vi "Basic Get Instruments Info.vi"() -> ()   [LabVIEW 2016]
doc: "Purpose: This example shows how to retrieve information about Fluigent instruments: type, controller, serial number, unique ID...\nHardware setup: At least one Fluigent pressure or sensor module"
uses:
  TypeDefs/fgt_INSTRUMENT_TYPE.ctl
  TypeDefs/fgt_CHANNEL_INFO.ctl
  TypeDefs/fgt_SENSOR_TYPE.ctl
  TypeDefs/fgt_CONTROLLER_INFO.ctl
  TypeDefs/fgt_VALVE_TYPE.ctl
  fgt_SDK.lvlib
panel:
  in  "Tab Control":T1(tab)
  out "Controllers channels info":T2[](array[typedef]) {"firmware" format="%04x"}
  out "Detected instruments":T4(array[cluster])
  out "Controllers count":i32
  out "Instruments count":i32
  out "Valve channels type":T5[](array[typedef])
  out "Valve channels count":u32
  out "Valve channels info":T6[](array[typedef]) {"firmware" format="%04x"}
  out "Pressure channels count":u32
  out "Sensor channels count":u32
  out "TTL channels count":u32
  out "Pressure channels info":T6[](array[typedef]) {"firmware" format="%04x"}
  out "Sensor channels info":T6[](array[typedef]) {"firmware" format="%04x"}
  out "Sensor channels type":T7[](array[typedef])
  out "TTL channels info":T6[](array[typedef]) {"firmware" format="%04x"}
  out "error out":errorcluster
  # "Hit the \"Run\" button to retrieve information about all Fluigent connected instruments"
  # "Hit the \"Run\" button to start the regulation"
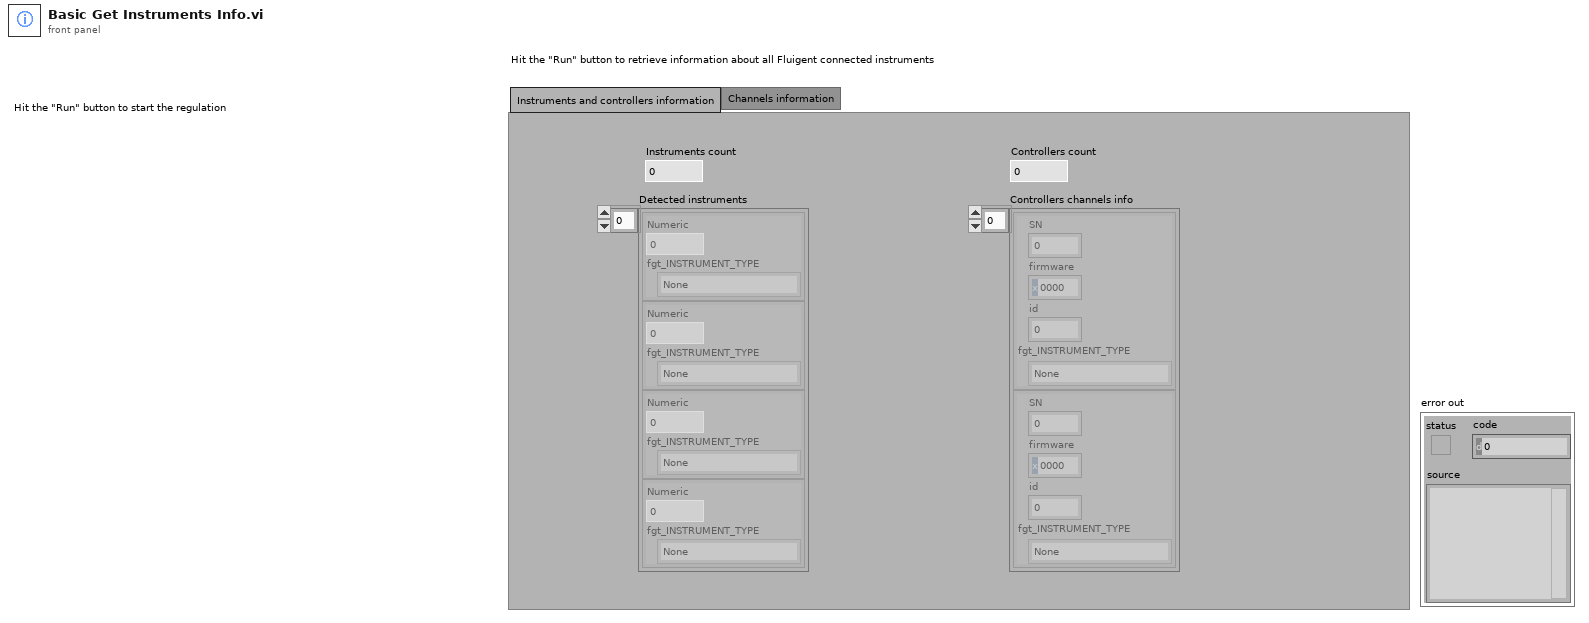
[diagram p1: front panel]
types:
  T1 = enum32{"Instruments and controllers information", "Channels information"}
  T2 = typedef "fgt_SDK.lvlib/fgt_CONTROLLER_INFO.ctl" = cluster{"SN":u16, "firmware":u16, "id":u32, "fgt_INSTRUMENT_TYPE":T3}
  T3 = typedef "fgt_SDK.lvlib/fgt_INSTRUMENT_TYPE.ctl" = enum32{"None", "MFCS", "MFCS_EZ", "FRP", "LineUP", "IPS"}
  T4 = cluster{"Numeric":u16, "fgt_INSTRUMENT_TYPE":T3}[]
  T5 = typedef "fgt_SDK.lvlib/fgt_VALVE_TYPE.ctl" = enum32{"None", "MSwitch", "TwoSwitch", "LSwitch", "PSwitch"}
  T6 = typedef "fgt_SDK.lvlib/fgt_CHANNEL_INFO.ctl" = cluster{"ControllerSN":u16, "firmware":u16, "DeviceSN":u16, "position":u32, "index":u32, "indexID":u32, "fgt_INSTRUMENT_TYPE":T3}
  T7 = typedef "fgt_SDK.lvlib/fgt_SENSOR_TYPE.ctl" = enum32{"None", "XS_single", "S_single", "S_dual", "M_single", "M_dual", "L_single", "L_dual", "XL_single", "Pressure_S", "Pressure_M", "Pressure_XL"}
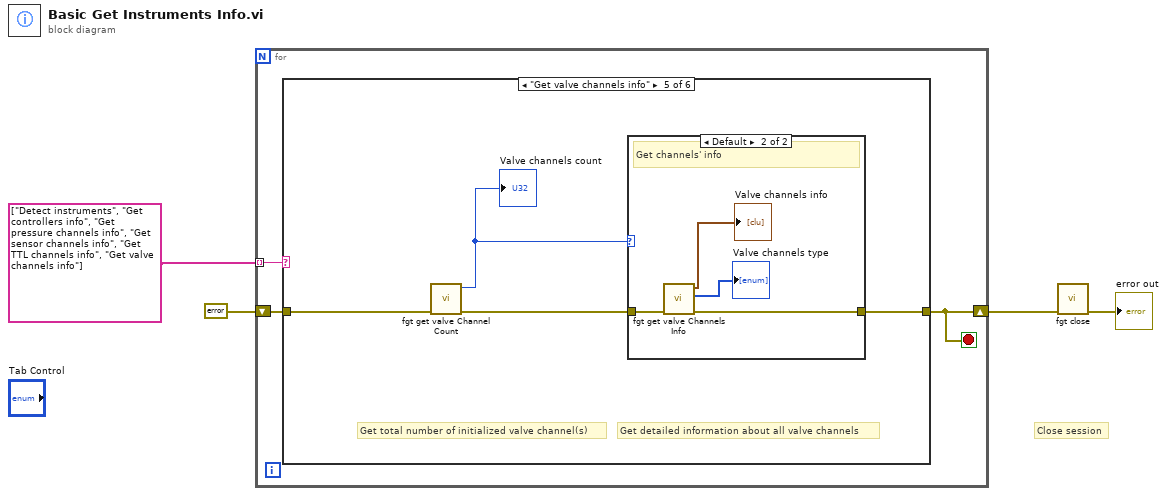
[diagram p0: block diagram]
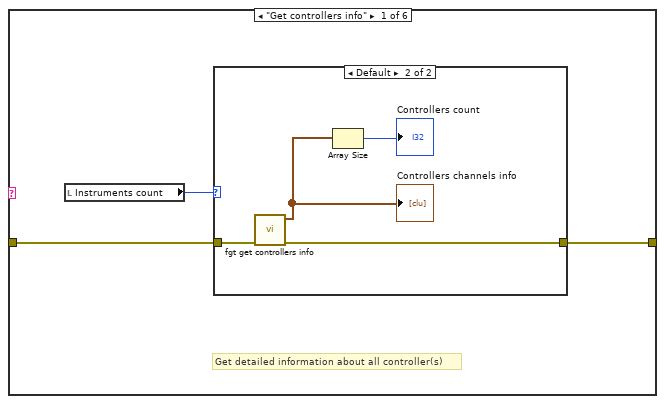
[diagram p2: hidden frame]
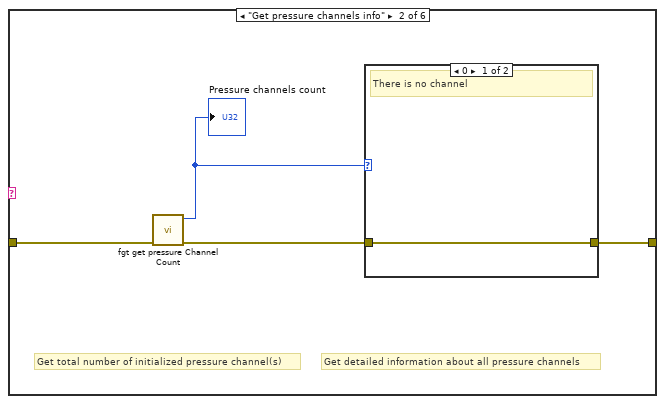
[diagram p4: hidden frame]
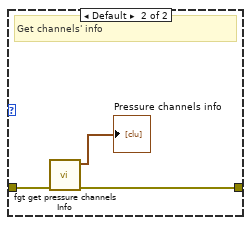
[diagram p5: hidden frame]
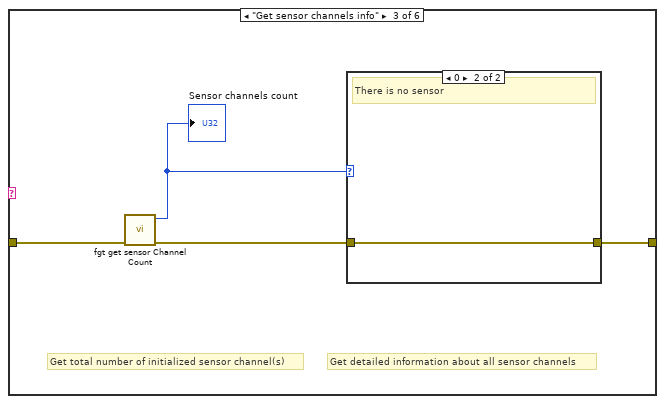
[diagram p6: hidden frame]
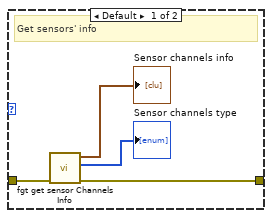
[diagram p7: hidden frame]
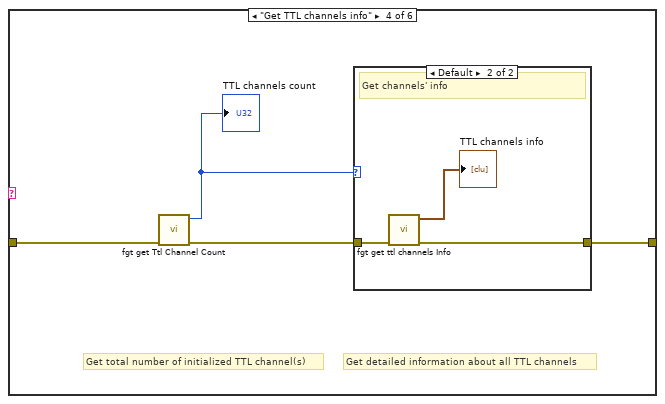
[diagram p8: hidden frame]
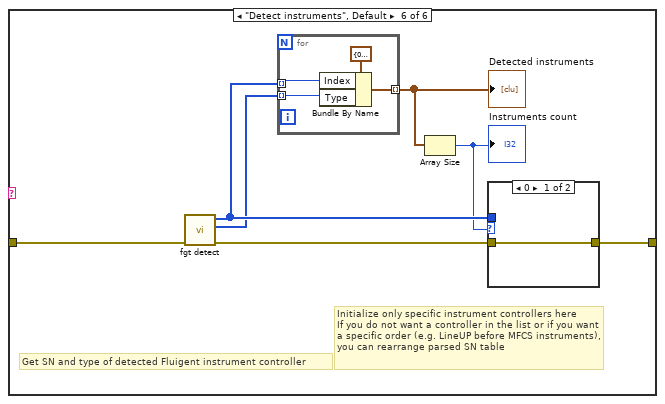
[diagram p11: hidden frame]
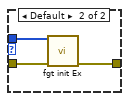
[diagram p12: hidden frame]
diagram:
  # "Close session"
  n1 = for {
    tunnel: string[] ["Detect instruments", "Get controllers info", "Get pressure channels info", "Get sensor channels info", "Get TTL channels info", "Get valve channels info"] -> [w7] mode=indexing
    shift-right: [w5] -> w1
    shift-left: errorcluster {"status"=FALSE, "code"=0, "source"=""} ("error in (no error)") -> [w6]
    stop <- w5 stop-if-true
    n2 = case shown="\"Get valve channels info\"" w7 {
      tunnel: [w9 w17 w25 w34 w44 w53] -> w5
      tunnel: w6 -> [w10 w18 w26 w35 w43 w52]
      frame "Get controllers info" {
        # "Get detailed information about all controller(s)"
        n3 = local read "Instruments count"() -> (w8:i32)
        n4 = case shown="Default" w8 {
          tunnel: w10 -> [w11 w15]
          tunnel: [w11 w14] -> w9
          frame 0 {
          }
          frame Default {
            n5 = call "fgt get controllers info.vi"("error in (no error)"=w15) -> ("error out"=w14:errorcluster, "Controllers channels info"=w12:T2[])  [unwired: 9 in]
            "Controllers channels info" <- w12
            n6 = Array Size(array=w12) -> (size(s)=→"Controllers count":i32)
          }
        }
      }
      frame "Get pressure channels info" {
        # "Get detailed information about all pressure channels"
        # "Get total number of initialized pressure channel(s)"
        n7 = call "fgt get pressure Channel Count.vi"("error in (no error)"=w18) -> ("error out"=w19:errorcluster, "nbPChan out"=w16:u32)  [unwired: 9 in]
        "Pressure channels count" <- w16
        n8 = case shown="0" w16 {
          tunnel: w19 -> [w20 w22]
          tunnel: [w20 w21] -> w17
          frame 0 {
            # "There is no channel"
          }
          frame Default {
            # "Get channels' info"
            n9 = call "fgt get pressure channels Info.vi"("error in (no error)"=w22) -> ("error out"=w21:errorcluster, "Pressure channels info"=→"Pressure channels info":T6[])  [unwired: 9 in]
          }
        }
      }
      frame "Get sensor channels info" {
        # "Get detailed information about all sensor channels"
        # "Get total number of initialized sensor channel(s)"
        n10 = call "fgt get sensor Channel Count.vi"("error in (no error)"=w26) -> ("error out"=w27:errorcluster, "nbSChan out"=w24:u32)  [unwired: 9 in]
        "Sensor channels count" <- w24
        n11 = case shown="0" w24 {
          tunnel: w27 -> [w29 w32]
          tunnel: [w28 w32] -> w25
          frame Default {
            # "Get sensors' info"
            n12 = call "fgt get sensor Channels Info.vi"("error in (no error)"=w29) -> ("error out"=w28:errorcluster, "Sensor channels type"=→"Sensor channels type":T7[], "Sensor channels info"=→"Sensor channels info":T6[])  [unwired: 8 in]
          }
          frame 0 {
            # "There is no sensor"
          }
        }
      }
      frame "Get TTL channels info" {
        # "Get detailed information about all TTL channels"
        # "Get total number of initialized TTL channel(s)"
        n13 = call "fgt get Ttl Channel Count.vi"("error in (no error)"=w35) -> ("error out"=w36:errorcluster, "nbTtlChan out"=w33:u32)  [unwired: 9 in]
        "TTL channels count" <- w33
        n14 = case shown="Default" w33 {
          tunnel: w36 -> [w37 w39]
          tunnel: [w37 w38] -> w34
          frame 0 {
            # "There is no channel"
          }
          frame Default {
            # "Get channels' info"
            n15 = call "fgt get ttl channels Info.vi"("error in (no error)"=w39) -> ("error out"=w38:errorcluster, "TTL channels info"=→"TTL channels info":T6[])  [unwired: 9 in]
          }
        }
      }
      frame "Get valve channels info" {
        # "Get detailed information about all valve channels"
        # "Get total number of initialized valve channel(s)"
        n16 = call "fgt get valve Channel Count.vi"("error in (no error)"=w43) -> ("error out"=w42:errorcluster, "nbVChan out"=w41:u32)  [unwired: 9 in]
        "Valve channels count" <- w41
        n17 = case shown="Default" w41 {
          tunnel: w42 -> [w45 w49]
          tunnel: [w45 w48] -> w44
          frame 0 {
            # "There is no channel"
          }
          frame Default {
            # "Get channels' info"
            n18 = call "fgt get valve Channels Info.vi"("error in (no error)"=w49) -> ("error out"=w48:errorcluster, "Valve channels type"=→"Valve channels type":T5[], "Valve channels info"=→"Valve channels info":T6[])  [unwired: 8 in]
          }
        }
      }
      frame "Detect instruments", Default {
        # "Initialize only specific instrument controllers here\nIf you do not want a controller in the list or if you want a specific order (e.g. LineUP before MFCS instruments), you can\trearrange parsed SN table"
        # "Get SN and type of detected Fluigent instrument controller"
        n19 = call "fgt detect.vi"("error in (no error)"=w52) -> ("error out"=w55:errorcluster, "type out"=w54:T3[], "SN out"=w56:u16[])  [unwired: 8 in]
        n20 = for {
          tunnel: w56 -> [w64] mode=indexing
          tunnel: w54 -> [w63] mode=indexing
          tunnel: [w62] -> w51 mode=indexing
          n21 = Bundle By Name(cluster=cluster{"Index":u16, "Type":T3} {"Index"=0, "Type"=enum."None"}, "Index"=w64, "Type"=w63) -> (w62:cluster{"Index":u16, "Type":T3})
        }
        "Detected instruments" <- w51
        n22 = Array Size(array=w51) -> (size(s)=w50:i32)
        "Instruments count" <- w50
        n23 = case shown="0" w50 {
          tunnel: w56 -> [_ w60]
          tunnel: w55 -> [w57 w59]
          tunnel: [w57 w58] -> w53
          frame 0 {
          }
          frame Default {
            n24 = call "fgt init Ex.vi"("error in (no error)"=w59, "SN"=w60) -> ("error out"=w58:errorcluster)  [unwired: 8 in, 1 out]
          }
        }
      }
    }
  }
  n25 = call "fgt close.vi"("error in (no error)"=w1) -> ("error out"=→"error out":errorcluster)  [unwired: 10 in]
